vi "Convert Channel Settings to PWM.vi"(11 "channel settings":T1[](array[typedef])) -> (1 "channel default values":dbl[](array[numeric]), 2 "channel names":string[](array[string]), 3 "PWM":T3 {"PWM Channels"."PWM frequency" items=["1 Hz", "50 Hz", "250 Hz", "500 Hz", "1 kHz", "5 kHz", "10 kHz", "20 kHz"]})   [LabVIEW 2020, in "Scan Engine Scripting.lvlib"]
uses:
  Scan Engine Scripting.lvlib
  Includes/Modules.lvlibp/SD Module/Type Defs/PWM.ctl
  Includes/Modules.lvlibp/SD Module/Type Defs/PWM Channel.ctl
  Modules/Mode Classes/Controls/pwm channel settings.ctl
  Modules/Channel Classes/PWM Output Channel/Frequency.ctl
  Includes/Modules.lvlibp/SD Module/SD Module.lvclass
  Modules/Channel Classes/PWM Output Channel/PWM Output Channel.lvclass
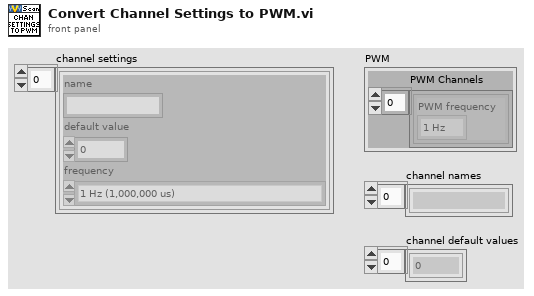
[diagram p1: front panel]
types:
  T1 = typedef "Scan Engine Scripting.lvlib/pwm channel settings.ctl" = cluster{"name":string, "default value":dbl, "frequency":T2}
  T2 = typedef "Scan Engine Scripting.lvlib/PWM Output Channel.lvclass/Frequency.ctl" = enum16{"1 Hz (1,000,000 us)", "50 Hz (20,000 us)", "250 Hz (4,000 us)", "500 Hz (2,000 us)", "1 kHz (1,000 us)", "5 kHz (200 us)", "10 kHz (100 us)", "20 kHz (50 us)"}
  T3 = typedef "Modules.lvlibp/SD Module.lvclass/PWM.ctl" = cluster{"PWM Channels":T4[]}
  T4 = typedef "Modules.lvlibp/SD Module.lvclass/PWM Channel.ctl" = cluster{"PWM frequency":u32}
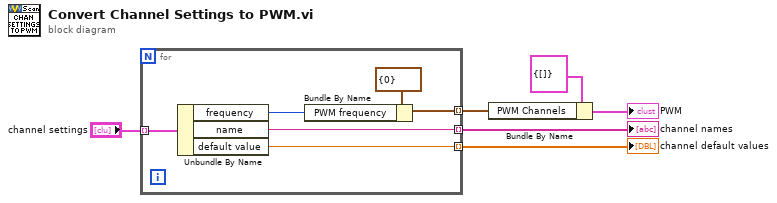
[diagram p0: block diagram]
diagram:
  n1 = for {
    tunnel: "channel settings" -> [w12] mode=indexing
    tunnel: [w11] -> w4 mode=indexing
    tunnel: [w10] -> w5 mode=indexing
    tunnel: [w9] -> w6 mode=indexing
    n2 = Unbundle By Name(w12) -> ("frequency"=w7:T2, "name"=w10:string, "default value"=w9:dbl)
    n3 = Bundle By Name(cluster=T4 {"PWM frequency"=0} ("PWM Channel"), "PWM frequency"=w7) -> (w11:T4)
  }
  "channel default values" <- w6
  "channel names" <- w5
  n4 = Bundle By Name(cluster=T3 {"PWM Channels"=[]} ("PWM"), "PWM Channels"=w4) -> (→"PWM":T3)
